vi "FdxCmdTMSubscriberControlCvi.vi"(8 "error in":errorcluster, 9 "SubscriberControlIn":T1, 10 "TMHandle":u32, 11 "InstrumentHandle":u32) -> (0 "error out":errorcluster, 2 "TMHandleOut":u32, 3 "InstrumentHandle":u32)   [LabVIEW 2020, in "AIM664LV.lvlib"]
doc: "This function is used to change the configuration of a subscriber with respect to a Time Manager. This function can be called while a Time Manager is running."
uses:
  AIM664LV.lvlib
  AFDX_LibraryAdmin/FdxGlobalDllPath.vi
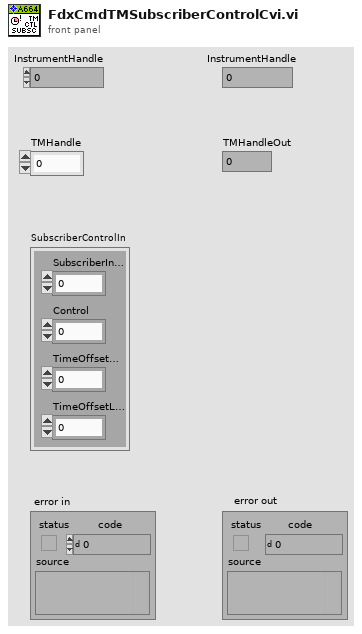
[diagram p1: front panel]
types:
  T1 = cluster{"SubscriberIndex":u8, "Control":u32, "TimeOffsetHighc":u16, "TimeOffsetLow":u32}
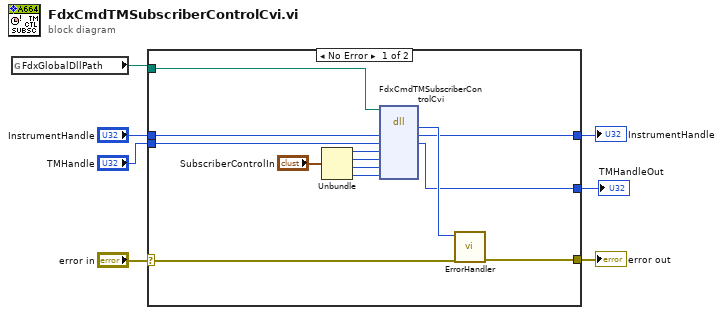
[diagram p0: block diagram]
diagram:
  n1 = global read "FdxGlobalDllPath.vi" "FdxGlobalDllPath"() -> (w5:path)
  n2 = case shown="No Error" "error in" {
    selector: "error in" -> [w19 w23]
    tunnel: [w20 w23] -> w7
    tunnel: w5 -> [w12 _]
    tunnel: "InstrumentHandle" -> [w11 w22]
    tunnel: [w10 w22] -> w3
    tunnel: "TMHandle" -> [w9 w21]
    tunnel: [w8 w21] -> w1
    frame No Error {
      n3 = Unbundle("SubscriberControlIn") -> ("SubscriberIndex"=w16:u8, "Control"=w15:u32, "TimeOffsetHighc"=w14:u16, "TimeOffsetLow"=w13:u32)
      n4 = dll-call lib="aim_fdx.19.dll" fn="FdxCmdTMSubscriberControlCvi" label="FdxCndTMSubscriberControlCvi"(path in=w12, "InstrumentHandle"=w11, "TMHandle"=w9, "SubscriberIndex"=w16, "Control"=w15, "TimeOffsetHigh"=w14, "TimeOffsetLow"=w13) -> ("status"=w18:i32, "InstrumentHandle"=w10:u32, "TMHandle"=w8:u32)  [unwired: 6 in, 2 out]
      n5 = call "ErrorHandler.vi"("error in"=w19, "AIM Error"=w18) -> ("error out"=w20:errorcluster)  [unwired: 9 in]
    }
    frame Error {
    }
  }
  "error out" <- w7
  "InstrumentHandle" <- w3
  "TMHandleOut" <- w1
